vi "Information.vi"(8 "error in (no error)":errorcluster, 9 "Context":T1, 10 "Information":refnum<class "Information.lvclass">, 11 "PID Controller in":refnum<class "PID Controller.lvclass">) -> (0 "error out":errorcluster, 3 "PID Controller out":refnum<class "PID Controller.lvclass">)   [LabVIEW 2021, in "PID Controller.lvclass"]
uses:
  Publish-Subscribe/Interfaces/Information/Information.lvclass
  Publish-Subscribe/Context.ctl
  PID Controller.lvclass
  PID Controller.lvclass/PID Controller.ctl
  <vilib>/addons/control/pid/NI_PID_pid.lvlib
  <vilib>/addons/control/pid/pid.llb/PID (DBL).vi
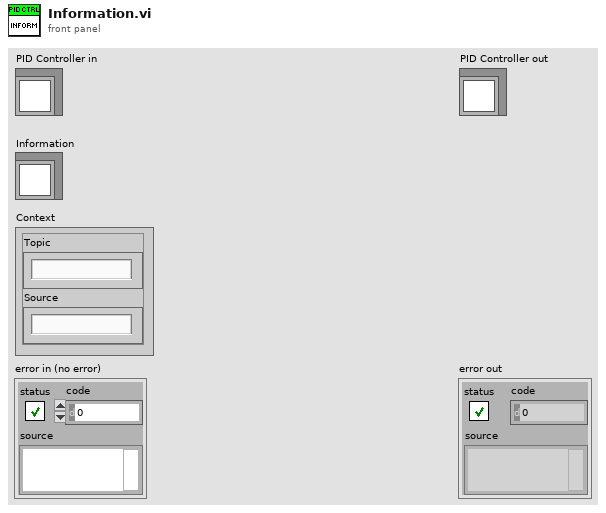
[diagram p1: front panel]
types:
  T1 = typedef "Context.ctl" = cluster{"Topic":string, "Source":string}
  T2 = typedef "PID Controller Configuration.ctl" = cluster{"P":dbl, "I":dbl, "D":dbl, "Set point":dbl, "Input instrument":string, "Output instrument":string}
  T3 = cluster{"proportional gain (Kc)":dbl, "integral time (Ti, min)":dbl, "derivative time (Td, min)":dbl}
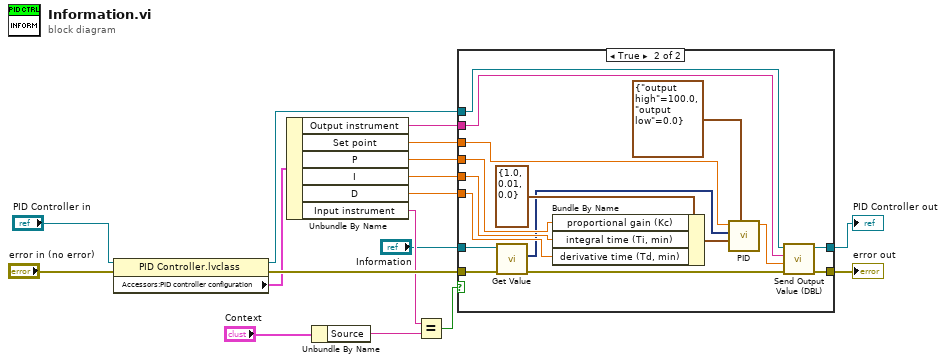
[diagram p0: block diagram]
diagram:
  n1 = property class="PID Controller.lvclass"(reference="PID Controller in", error in="error in (no error)") -> (reference out=w8:refnum<class "PID Controller.lvclass">, error out=w12:errorcluster, "Accessors:PID controller configuration"=w11:T2)
  n2 = Unbundle By Name(w11) -> ("Output instrument"=w17:string, "Set point"=w13:dbl, "P"=w14:dbl, "I"=w15:dbl, "D"=w16:dbl, "Input instrument"=w10:string)
  n3 = Unbundle By Name("Context") -> ("Source"=w4:string)
  n4 = Equal?(x=w10, y=w4) -> (x = y?=w9:bool)
  n5 = case shown="True" w9 {
    tunnel: w8 -> [w19 w29]
    tunnel: [w19 w28] -> w3
    tunnel: w12 -> [w18 w20]
    tunnel: w13 -> [_ w33]
    tunnel: w14 -> [_ w32]
    tunnel: w15 -> [_ w31]
    tunnel: w16 -> [_ w30]
    tunnel: [w18 w26] -> w2
    tunnel: w17 -> [_ w27]
    tunnel: "Information" -> [_ w23]
    frame False {
    }
    frame True {
      n6 = call-dynamic "Get Value.vi"("error in (no error)"=w20, "Information in"=w23) -> ("error out"=w21:errorcluster, "Value"=w22:dynamicdata)  [unwired: 7 in, 1 out]
      n7 = Bundle By Name(cluster=T3 {"proportional gain (Kc)"=1.0, "integral time (Ti, min)"=0.01, "derivative time (Td, min)"=0.0} ("PID gains"), "proportional gain (Kc)"=w32, "integral time (Ti, min)"=w31, "derivative time (Td, min)"=w30) -> (w34:T3)
      n8 = call-poly <vilib>:"PID.vi"("output range"=cluster{"output high":dbl, "output low":dbl} {"output high"=100.0, "output low"=0.0}, "PID gains"=w34, "process variable"=w22, "setpoint"=w33) -> ("output"=w24:dbl)  [unwired: 6 in, 1 out]
      n9 = call-dynamic "Send Output Value (DBL).vi"("error in (no error)"=w21, "DBL Value"=w24, "Name"=w27, "Template Module in"=w29) -> ("error out"=w26:errorcluster, "Template Module out"=w28:refnum<class "PID Controller.lvclass">)  [unwired: 6 in]
    }
  }
  "error out" <- w2
  "PID Controller out" <- w3
